vi "Configure Trigger.vi"(0 "VISA resource name":refnum<visa-resource-name>, 1 "Source (Immediate)":u16(ring) items=["Immediate", "Timer", "Manual", "Bus", "External"], 2 "Timer Delay (0.001 s)":dbl=0.001, 3 "Count Mode (Infinite)":u16(ring) items=["Infinite", "Custom Count"], 4 "Custom Count (1)":i32=1, 5 "error in":errorcluster, 6 "Auto Delay? (Custom)":bool, 8 "Delay (0 s)":dbl, 10 "Inititiate Mode (Init Continuous)":i16(ring)=1 items=["Don't Initiate"=-1, "Initiate Single"=0, "Initiate Continuous"=1]) -> (14 "VISA resource name out":refnum<visa-resource-name>, 19 "error out":errorcluster)   [LabVIEW 2016, in "Keithley 2182A.lvlib"]
uses:
  <instrlib>/Keithley 2182A/Keithley 2182A.lvlib
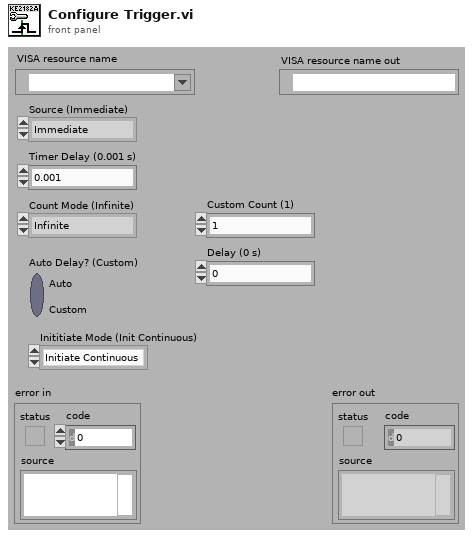
[diagram p1: front panel]
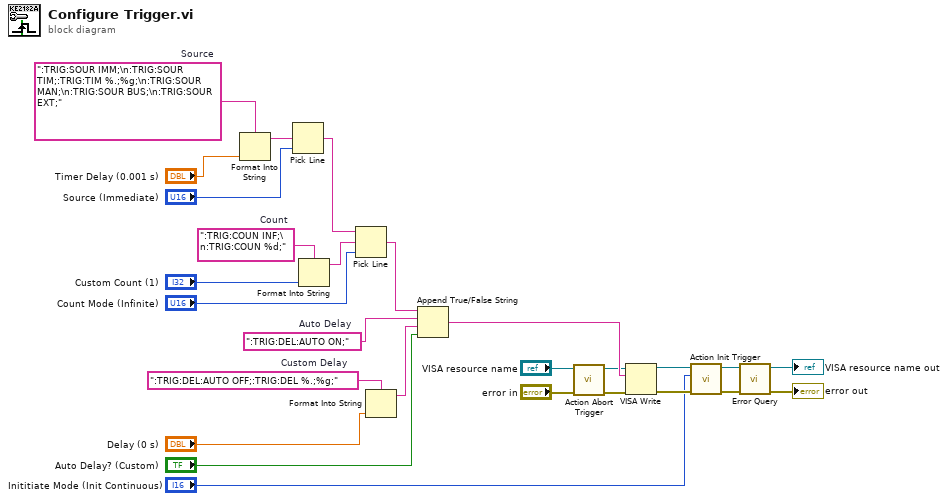
[diagram p0: block diagram]
diagram:
  w21 = ":TRIG:DEL:AUTO ON;"  # Auto Delay
  w18 = ":TRIG:DEL:AUTO OFF;:TRIG:DEL %.;%g;"  # Custom Delay
  w13 = ":TRIG:COUN INF;\n:TRIG:COUN %d;"  # Count
  w24 = ":TRIG:SOUR IMM;\n:TRIG:SOUR TIM;:TRIG:TIM %.;%g;\n:TRIG:SOUR MAN;\n:TRIG:SOUR BUS;\n:TRIG:SOUR EXT;"  # Source
  n1 = Format Into String(format string=w24, "Timer Delay (0.001 s)") -> (resulting string=w26:string)  [unwired: 2 in, 1 out]
  n2 = Pick Line(multi-line string=w26, line index="Source (Immediate)") -> (output string=w15:string)  [unwired: 1 in]
  n3 = Format Into String(format string=w13, "Custom Count (1)") -> (resulting string=w14:string)  [unwired: 2 in, 1 out]
  n4 = Pick Line(string ("")=w15, multi-line string=w14, line index="Count Mode (Infinite)") -> (output string=w22:string)
  n5 = Format Into String(format string=w18, "Delay (0 s)") -> (resulting string=w20:string)  [unwired: 2 in, 1 out]
  n6 = Append True/False String(1:"Auto Delay? (Custom)", 2:w20, 3:w21, 4:w22) -> (0:w27:string)
  n7 = call <instrlib>:"Action Abort Trigger.vi"("error in"="error in", "VISA resource name"="VISA resource name") -> ("error out"=w9:errorcluster, "VISA resource name out"=w8:refnum<visa-resource-name>)  [unwired: 8 in]
  n8 = VISA Write(VISA resource name=w8, write buffer=w27, error in (no error)=w9) -> (VISA resource name out=w6:refnum<visa-resource-name>, error out=w7:errorcluster)  [unwired: 1 out]
  n9 = call <instrlib>:"Action Init Trigger.vi"("error in"=w7, "Inititiate Mode (Init Continuous)"="Inititiate Mode (Init Continuous)", "VISA resource name"=w6) -> ("error out"=w4:errorcluster, "VISA resource name out"=w3:refnum<visa-resource-name>)  [unwired: 7 in]
  n10 = call <instrlib>:"Error Query.vi"("error in (no error)"=w4, "VISA resource name"=w3) -> ("error out"=→"error out":errorcluster, "VISA resource name out"=→"VISA resource name out":refnum<visa-resource-name>)  [unwired: 6 in, 2 out]
